vi "SetCommand.vi"(0 "MCU in":refnum<class "MCU.lvclass">, 1 "Device Code":T2, 5 "Parameter 1":string, 7 "Parameter 2":string, 9 "Parameter 3":string, 11 "error in (no error)":errorcluster, 12 "Command Code":T1) -> (4 "MCU out":refnum<class "MCU.lvclass">, 6 "Command":string, 15 "error out":errorcluster)   [LabVIEW 2020, in "MCU.lvclass"]
doc: "It creats a command concatenating the given parameters. According to the device, it would send the command through the corresponding communication bus."
uses:
  MCU.lvclass
  Controls/Device Code.ctl
  Controls/Device Command Code.ctl
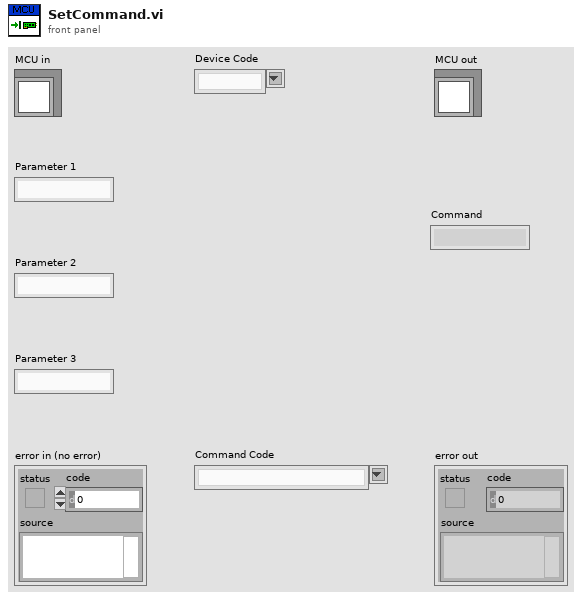
[diagram p1: front panel]
types:
  T1 = typedef "Device Command Code.ctl" = string
  T2 = typedef "Device Code.ctl" = string
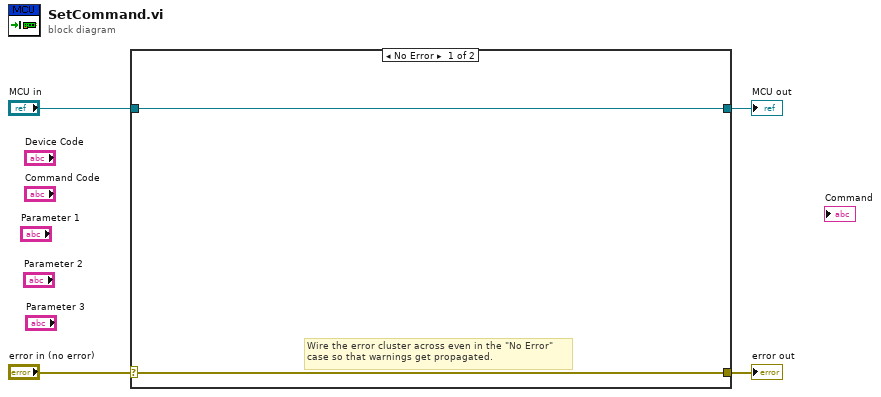
[diagram p0: block diagram]
diagram:
  n1 = case shown="No Error" "error in (no error)" {
    selector: "error in (no error)" -> [w5 w8]
    tunnel: [w5 w8] -> w3
    tunnel: [w6 w7] -> w1
    tunnel: "MCU in" -> [w6 w7]
    frame No Error {
      # "Wire the error cluster across even in the \"No Error\"\ncase so that warnings get propagated."
    }
    frame Error {
    }
  }
  "error out" <- w3
  "MCU out" <- w1
